vi "Measure all pixels on cell and save data.vi"(0 "Cell details cluster in":T3={"Measure?"=TRUE, "Area (cm^2)"=0.0, "Cell Label"="", "Cell Description"="", "Cell Position"=0, "Time in rig (s)"=0.0, "Time to next scan (s)"=0.0, "Scan number"=0.0, "When did you stick it in?"=0.0, "Time between scans (s)"=0.0, "Time of the last scan (s)"=0.0, "Scan settings in queue"=0, "Sample Holder"=0.0, "User Name"=""} {"Scan settings in queue" items=["Regular", "Inverted", "MartinaSettings"]; "Time of the last scan (s)" format="%<%H:%M:%S>t"; "When did you stick it in?" format="%<%H:%M:%S>t"; "Time to next scan (s)" format="%<%H:%M:%S>t"; "Time in rig (s)" format="%<%H:%M:%S>t"}, 1 "Username":string, 5 "Cell Description":string, 6 "JV Refnum":refnum<vi>, 7 "Cell position":dbl, 8 "Tbl Refnum":refnum<vi>, 9 "Sample Holder":dbl, 11 "Scan settings in queue":dbl, 12 "Scan settings array":T1 {"Number of pixels to stabilize \nper substrate" items=["1", "2", "3", "4", "5", "6", "7", "8"]; "Range Options" items=["Auto Range", "Semi-Auto Range", "100 uA", "1 mA", "10 mA", "100 mA", "1A"]}, 13 "Time Zero":timestamp, 14 "Jt Refnum":refnum<vi>) -> (4 "Cell details cluster out":T3={"Measure?"=TRUE, "Area (cm^2)"=0.0, "Cell Label"="", "Cell Description"="", "Cell Position"=0, "Time in rig (s)"=0.0, "Time to next scan (s)"=0.0, "Scan number"=0.0, "When did you stick it in?"=0.0, "Time between scans (s)"=0.0, "Time of the last scan (s)"=0.0, "Scan settings in queue"=0, "Sample Holder"=0.0, "User Name"=""} {"Scan settings in queue" items=["Regular", "Inverted", "MartinaSettings"]; "Time of the last scan (s)" format="%<%H:%M:%S>t"; "When did you stick it in?" format="%<%H:%M:%S>t"; "Time to next scan (s)" format="%<%H:%M:%S>t"; "Time in rig (s)" format="%<%H:%M:%S>t"}, 10 "Jt Curve":cluster{"Y":dbl[], "Y":dbl[]}[](graph) caption="JV Curve", 15 "JV curve image path":path)   [LabVIEW 2011]
uses:
  Typedefs/Queue cluster.ctl
  Typedefs/Scan settings array.ctl
  Typedefs/Scan settings.ctl
  <instrlib>/keithley_24xx/Keithley 24XX/Keithley 24XX.lvlib
panel:
  out "File path for master log":path
  out "File path for device log":path
  in  "Tab Control 4":enum32{"Page 1"}(tab)
  out "JV Curve":cluster{"Y":dbl[], "Y":dbl[]}[](graph)
  in  "VISA resource name":refnum<visa-resource-name>="GPIB0::24::INSTR"
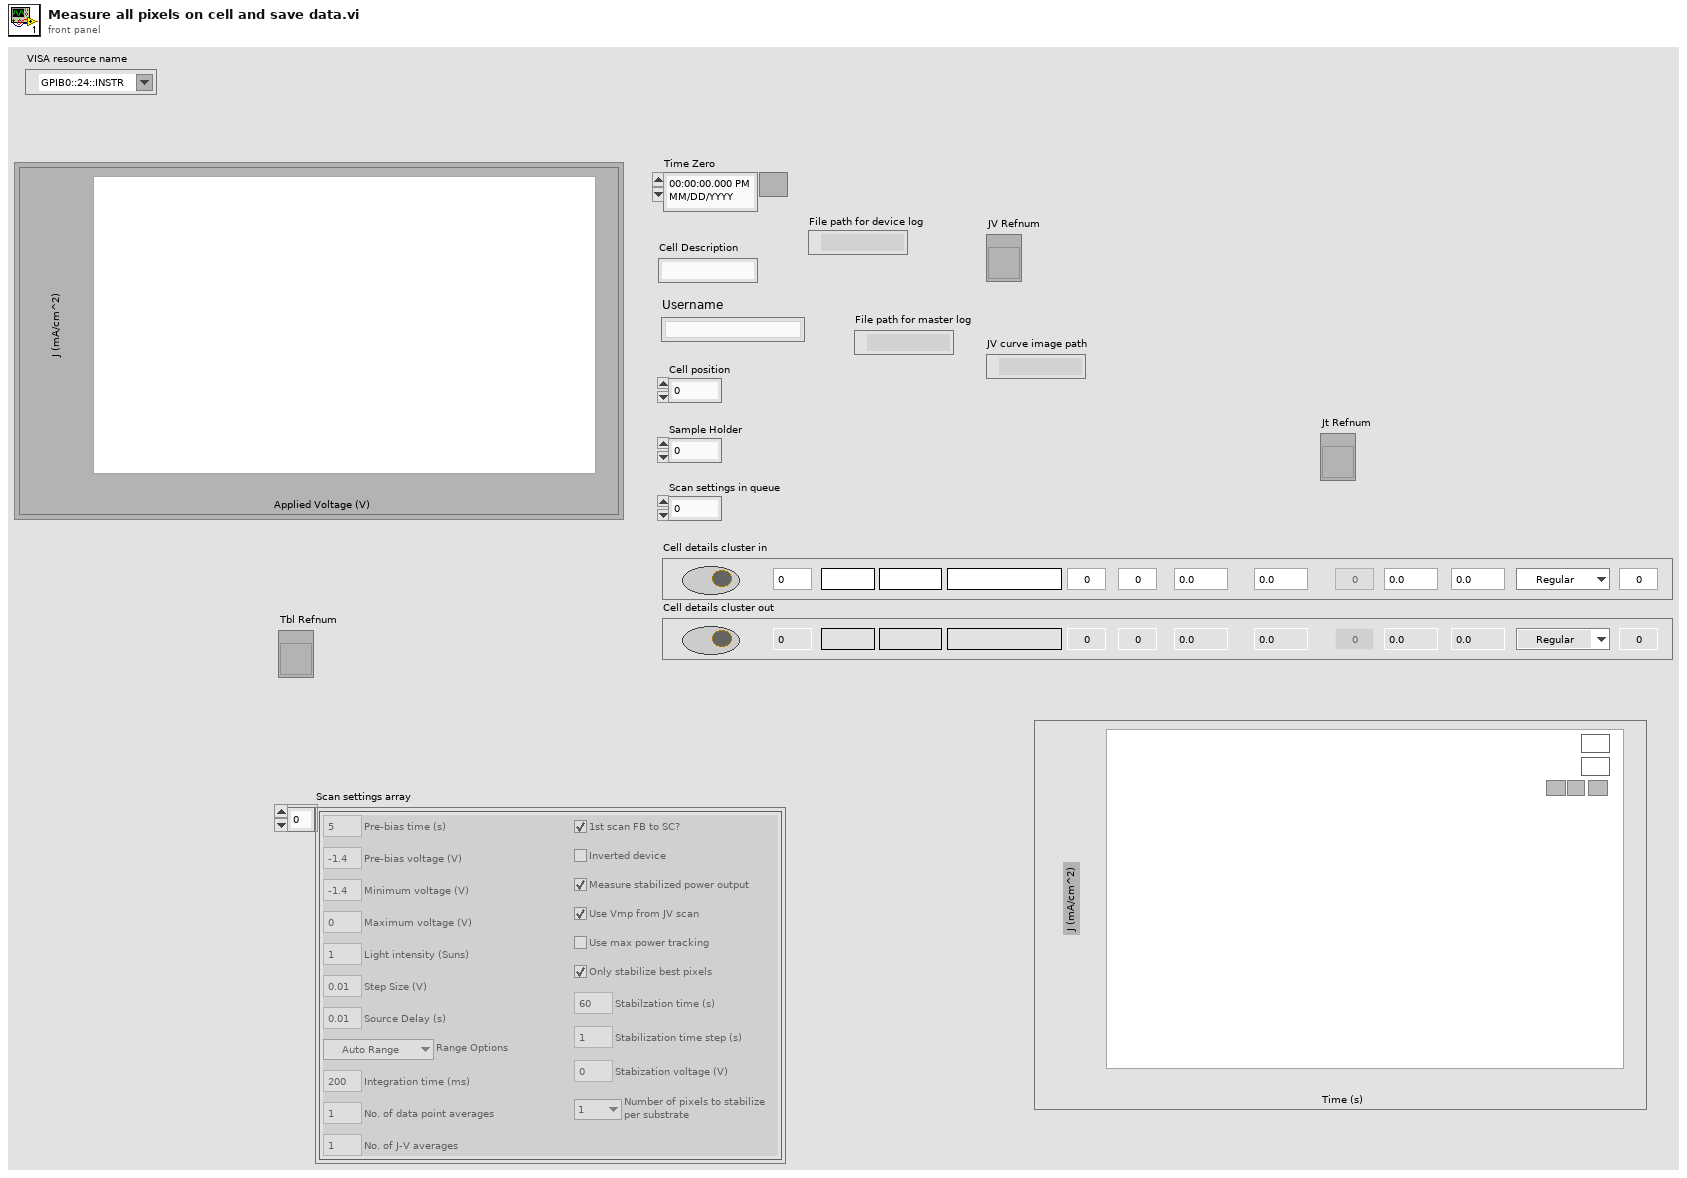
[diagram p1: front panel]
types:
  T1 = typedef "Scan settings array.ctl" = T2[]
  T2 = typedef "Scan settings.ctl" = cluster{"Light intensity (Suns)":dbl, "Pre-bias time (s)":dbl, "Maximum voltage (V)":dbl, "Minimum voltage (V)":dbl, "Range Options":u16, "1st scan FB to SC?":bool, "Step Size (V)":dbl, "Source Delay (s)":dbl, "Inverted device":bool, "Measure stabilized power output":bool, "Stabilzation time (s)":dbl, "Use Vmp from JV scan":bool, "Stabization voltage (V)":dbl, "Only stabilize best pixels":bool, "Number of pixels to stabilize \nper substrate":u16, "Stabilization time step (s)":dbl, "Use max power tracking":bool, "Pre-bias voltage (V)":dbl, "No. of data point averages":dbl, "No. of J-V averages":dbl, "Integration time (ms)":dbl}
  T3 = typedef "Queue cluster.ctl" = cluster{"Measure?":bool, "Area (cm^2)":dbl, "Cell Label":string, "Cell Description":string, "Cell Position":i32, "Time in rig (s)":dbl, "Time to next scan (s)":dbl, "Scan number":dbl, "When did you stick it in?":dbl, "Time between scans (s)":dbl, "Time of the last scan (s)":dbl, "Scan settings in queue":u16, "Sample Holder":dbl, "User Name":string}
  T4 = typedef "imagedata.ctl" = cluster{"image type":i32, "image depth":i32, "image":u8[], "mask":u8[], "colors":u32[], "Rectangle":cluster{"left":i16, "top":i16, "right":i16, "bottom":i16}}
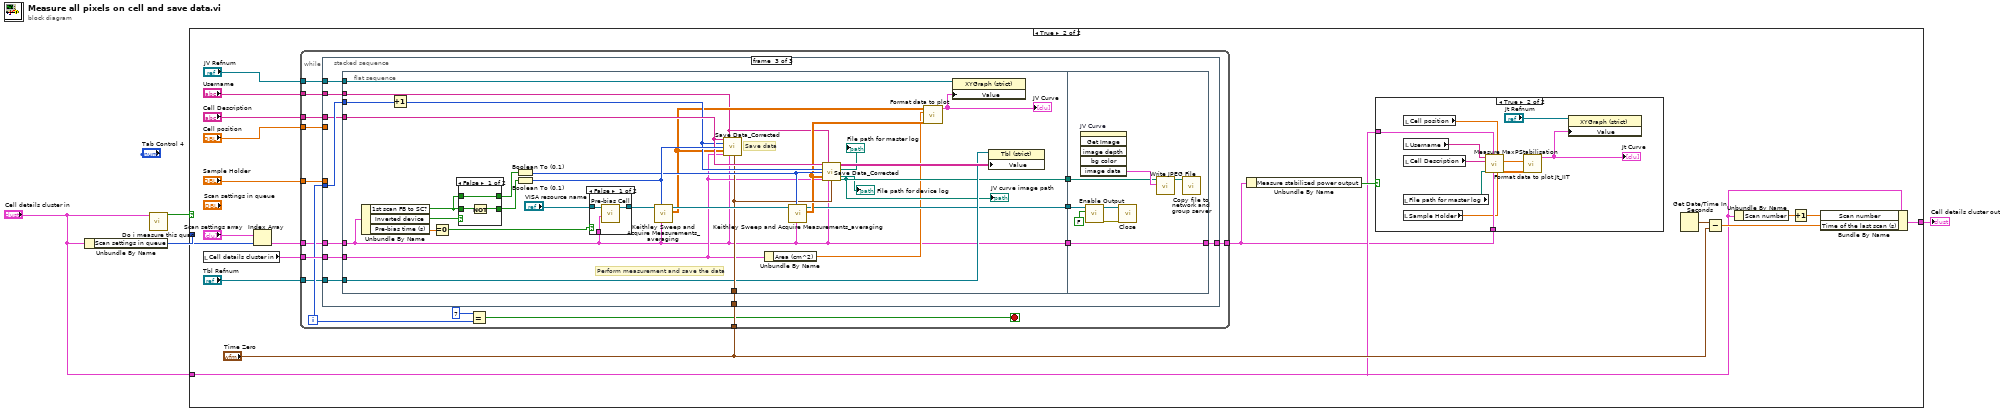
[diagram p0: block diagram]
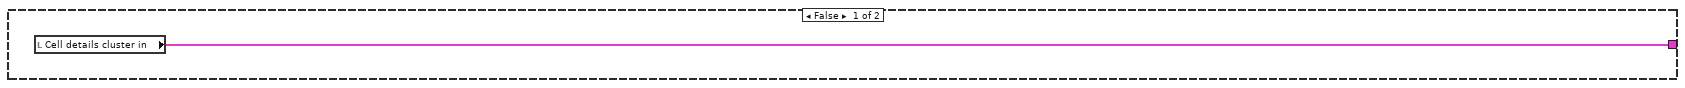
[diagram p2: hidden frame]
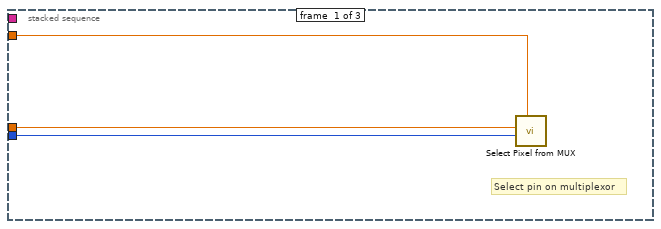
[diagram p4: hidden frame]
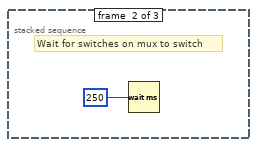
[diagram p5: hidden frame]
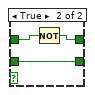
[diagram p7: hidden frame]
diagram:
  n1 = Unbundle By Name("Cell details cluster in") -> ("Scan settings in queue"=w1:u16)
  n2 = call "Do i measure this quad.vi"("Cell details"="Cell details cluster in") -> ("Measure cell?"=w4:bool)  [unwired: 10 in]
  n3 = case shown="True" w4 {
    tunnel: [w5 w15] -> w3
    tunnel: "Cell details cluster in" -> [_ w10]
    tunnel: w1 -> [_ w6]
    frame False {
      n4 = local read "Cell details cluster in"() -> (w5:T3)
    }
    frame True {
      n5 = local read "Cell details cluster in"() -> (w20:T3)
      n6 = Index Array(array="Scan settings array", index=w6) -> (element=w7:T2)
      n7 = while {
        tunnel: w20 -> [w48]
        tunnel: "Cell position" -> [w47]
        tunnel: "Sample Holder" -> [w44]
        tunnel: "Cell Description" -> [w43]
        tunnel: "Time Zero" -> [w42]
        tunnel: "Username" -> [w40]
        tunnel: "JV Refnum" -> [w39]
        tunnel: "Tbl Refnum" -> [w38]
        tunnel: w7 -> [w37]
        tunnel: [w36] -> w9
        i -> [w45]
        stop <- w41 stop-if-true
        n8 = stacked-sequence {
          tunnel: w48 -> [_ _ w62]
          tunnel: w47 -> [w49 _ _]
          tunnel: w45 -> [w50 _ w64]
          tunnel: w44 -> [w51 _ _]
          tunnel: w43 -> [_ _ w63]
          tunnel: w42 -> [_ _ w61]
          tunnel: w40 -> [_ _ w60]
          tunnel: w39 -> [_ _ w59]
          tunnel: w38 -> [_ _ w58]
          tunnel: w37 -> [_ _ w55]
          tunnel: [_ _ w54] -> w36
          frame #0 {
            # "Select pin on multiplexor"
            n9 = call "Select Pixel from MUX.vi"("Cell position"=w49, "Pixel"=w50, "Sample Holder"=w51) -> ()  [unwired: 9 in]
          }
          frame #1 {
            # "Wait for switches on mux to switch"
            n10 = Wait (ms)(milliseconds to wait=250) -> ()  [unwired: 1 out]
          }
          frame #2 {
            n11 = flat-sequence {
              tunnel: w64 -> [w92]
              tunnel: w63 -> [w90]
              tunnel: w62 -> [w69]
              tunnel: w61 -> [w87]
              tunnel: w60 -> [w84]
              tunnel: w59 -> [w83]
              tunnel: w58 -> [w81]
              tunnel: [w79] -> w57
              tunnel: [w78] -> w56
              tunnel: w55 -> [w65]
              tunnel: [w65] -> w53
              tunnel: w57 -> [w110]
              tunnel: w56 -> [w106]
              tunnel: [w104] -> w54
              tunnel: w53 -> [w104]
              frame #0 {
                # "Perform measurement and save the data"
                # "Save data"
                n12 = Unbundle By Name(w65) -> ("1st scan FB to SC?"=w67:bool, "Inverted device"=w66:bool, "Pre-bias time (s)"=w73:dbl)
                n13 = Increment(x=w92) -> (x+1=w89:i32)
                n14 = Equal To 0?(x=w73) -> (x = 0?=w72:bool)
                n15 = case shown="False" w66 {
                  tunnel: [w99 w103] -> w76
                  tunnel: w67 -> [w100 w103]
                  tunnel: w67 -> [w98 w102]
                  tunnel: [w98 w101] -> w75
                  frame False {
                    n16 = Not(x=w100) -> (.not. x?=w99:bool)
                  }
                  frame True {
                    n17 = Not(x=w102) -> (.not. x?=w101:bool)
                  }
                }
                n18 = Boolean To (0,1)(Boolean=w75) -> (0, 1=w88:i16)
                n19 = Boolean To (0,1)(Boolean=w76) -> (0, 1=w93:i16)
                n20 = case shown="False" w72 {
                  tunnel: "VISA resource name" -> [w96 w97]
                  tunnel: [w95 w97] -> w70
                  tunnel: w65 -> [w94 _]
                  frame False {
                    n21 = call "Pre-bias Cell.vi"("Scan Settings JV"=w94, "VISA resource name"=w96) -> ("VISA resource name out"=w95:refnum<visa-resource-name>)  [unwired: 8 in, 1 out]
                  }
                  frame True {
                  }
                }
                n22 = call "Keithley Sweep and Acquire Measurements_averaging.vi"("Scan Settings JV"=w65, "Sweep Direction"=w93, "VISA resource name"=w70) -> ("Data Array"=w86:dbl[][], "VISA resource name out"=w91:refnum<visa-resource-name>)  [unwired: 7 in]
                n23 = call "Save Data_Corrected.vi"("Experiment Indicator"=w90, "Username"=w84, "Pixel"=w89, "Scan direction"=w93, "Data Array"=w86, "Cell details cluster"=w69, "Show me Scan \nSettings JV set"=w65, "Time zero"=w87) -> ()  [unwired: 1 in, 7 out]
                n24 = Unbundle By Name(w69) -> ("Area (cm^2)"=w68:dbl)
                n25 = call "Keithley Sweep and Acquire Measurements_averaging.vi"("Scan Settings JV"=w65, "Sweep Direction"=w88, "VISA resource name"=w91) -> ("Data Array"=w85:dbl[][], "VISA resource name out"=w78:refnum<visa-resource-name>)  [unwired: 7 in]
                n26 = call "Save Data_Corrected.vi"("Experiment Indicator"=w90, "Username"=w84, "Pixel"=w89, "Scan direction"=w88, "Data Array"=w85, "Cell details cluster"=w69, "Show me Scan \nSettings JV set"=w65, "Time zero"=w87) -> ("Master Log"=w82:string[][], "File path for master log"=→"File path for master log":path, "File path for device log"=→"File path for device log":path, "File path for JV image"=w79:path)  [unwired: 1 in, 3 out]
                "JV curve image path" <- w79
                n27 = call "Format data to plot.vi"("Data Array 2"=w85, "Device area (cm^2)"=w68, "Data Array"=w86) -> ("JV Curve"=w80:cluster{"Y":dbl[], "Y":dbl[]}[])  [unwired: 8 in]
                "JV Curve" <- w80
                n28 = property class="XYGraph (strict)"(reference=w83, "Value"=w80) -> ()  [unwired: 1 in, 2 out]
                n29 = property class="Tbl (strict)"(reference=w81, "Value"=w82) -> ()  [unwired: 1 in, 2 out]
              }
              frame #1 {
                n30 = invoke on="JV Curve" class="XYGraph (strict)" method="Get Image"() -> ("image data"=w111:T4)  [unwired: 6 in, 5 out]
                n31 = call <instrlib>:"Enable Output.vi"("Enable Output (T: Enable)"=FALSE, "VISA resource name"=w106) -> ("error out"=w108:errorcluster, "VISA resource name out"=w107:refnum<visa-resource-name>)  [unwired: 8 in]
                n32 = call <instrlib>:"Close.vi"("error in (no error)"=w108, "VISA resource name"=w107) -> ()  [unwired: 9 in, 1 out]
                n33 = call <vilib>:"Write JPEG File.vi"("image data"=w111, "path to JPEG file"=w110) -> ("path"=w105:path)  [unwired: 8 in, 1 out]
                n34 = call "Copy file to network and group server.vi"("File path in"=w105) -> ()  [unwired: 10 in, 1 out]
              }
            }
          }
        }
        n35 = Equal?(x=7, y=w45) -> (x = y?=w41:bool)
      }
      n36 = Unbundle By Name(w9) -> ("Measure stabilized power output"=w11:bool)
      n37 = case shown="True" w11 {
        tunnel: w9 -> [_ w35]
        tunnel: w10 -> [_ w34]
        frame False {
        }
        frame True {
          n38 = local read "File path for master log"() -> (w29:path)
          n39 = local read "Sample Holder"() -> (w30:dbl)
          n40 = local read "Cell position"() -> (w31:dbl)
          n41 = local read "Username"() -> (w33:string)
          n42 = local read "Cell Description"() -> (w32:string)
          n43 = call "Measure MaxPStabilisation.vi"("Sample Holder"=w30, "Cell position"=w31, "Scan Settings JV"=w35, "Cell details cluster in"=w34, "File path of master log"=w29, "Experiment Title"=w32, "User Name"=w33) -> ("Data Array"=w27:dbl[][], "Area (cm^2)"=w28:dbl)  [unwired: 2 in, 1 out]
          n44 = call "Format data to plot Jt_IIT.vi"("Data Array 2"=w27, "Device Area (cm^2)"=w28) -> ("JV Curve"=w25:cluster{"Y":dbl[], "Y":dbl[]}[])  [unwired: 9 in]
          "Jt Curve" <- w25
          n45 = property class="XYGraph (strict)"(reference="Jt Refnum", "Value"=w25) -> ()  [unwired: 1 in, 2 out]
        }
      }
      n46 = Get Date/Time In Seconds() -> (seconds since 1Jan1904=w19:timestamp)
      n47 = Subtract(x=w19, y="Time Zero") -> (x-y=w14:dbl)
      n48 = Unbundle By Name(w10) -> ("Scan number"=w16:dbl)
      n49 = Increment(x=w16) -> (x+1=w17:dbl)
      n50 = Bundle By Name(cluster=w10, "Scan number"=w17, "Time of the last scan (s)"=w14) -> (w15:T3)
    }
  }
  "Cell details cluster out" <- w3
